vi "AerotechController.vi"() -> ()   [LabVIEW 2009]
uses:
  Controls/AerotechState.ctl
  Controls/AerotechCommand.ctl
  Controls/AerotechTarget.ctl
  Controls/AerotechScope.ctl
panel:
  out "Position error":dbl
  in  "Track threshold":dbl=5e-05
  in  "Gain [/s]":dbl=0.5
  out "Position":dbl
  out "State":T1
  in  "PROCESS":string="AEROTECH"
  in  "lpsParam":path=path "C:/OhanaOS/Instruments/Aerotech/Data/122764-A-1-1.prm"
  in  "lpsFirm":path=path "C:/u500/mmi/U500pci.jwp"
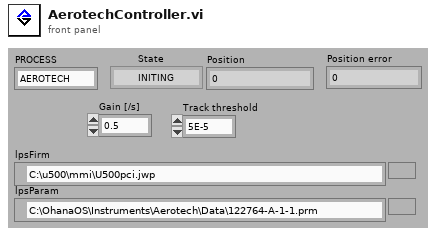
[diagram p1: front panel]
types:
  T1 = typedef "AerotechState.ctl" = enum16{"INITING", "IDLING", "SLEWING", "TRACKING", "MOVING", "HOMING", "STOPPING", "RECORDING"}
  T2 = typedef "AerotechCommand.ctl" = enum16{"TRACK", "POSITION", "STOP", "HOME", "QUIT", "RECORD"}
  T3 = typedef "AerotechSynchro.ctl" = cluster{"Command":refnum<queue>, "State":refnum<notifier>, "Target":refnum<notifier>, "Actual":refnum<notifier>, "Scope":refnum<notifier>}
  T4 = typedef "AerotechTarget.ctl" = cluster{"Time":timestamp, "Position":dbl, "Velocity":dbl}
  T5 = typedef "AerotechScope.ctl" = cluster{"First element":i32, "Buffer":i32[]}
  T6 = enum8{"Kill, clear memory", "Feedback Actual velocity data", "Feedback Command velocity data", "Feedback Auxiliary data", "Set time base (ms)", "Enable Tracking", "Stop Tracking, but keep data", "Set # of samples [1-2500]", "Set auxiliary sample type", "Feedback Auto tune Velocity", "Feedback Auto tune Torque"}
  T7 = cluster{"Position error":bool, "RMS current error":bool, "Integral error":bool, "Hardware limit +":bool, "Hardware limit -":bool, "Software limit +":bool, "Software limit -":bool, "Driver fault":bool, "Feedback device error":bool, "Global abort active":bool, "Velocity error":bool, "Feedrate > max setting error":bool, "Emergency stop":bool, "Driver interlock open":bool}
  T8 = cluster{"Axis 1 active":bool, "Axis 2 active":bool, "Axis 3 active":bool, "Axis 4 active":bool, "Axis 1 not in position":bool, "Axis 2 not in position":bool, "Axis 3 not in position":bool, "Axis 4 not in position":bool, "Plane 1 comm. busy":bool, "Plane 2 comm. busy":bool, "Plane 4 comm. busy":bool, "Plane 3 comm. busy":bool, "Queue 1 buffer not empty":bool, "Queue 2 buffer not empty":bool, "Queue 3 buffer not empty":bool, "Queue 4 buffer not empty":bool, "Plane 1 halted":bool, "Plane 2 halted":bool, "Plane 3 halted":bool, "Plane 4 halted":bool, "Global abort active":bool, "Feedhold active":bool, "PC Bus Interrupt high":bool, "Not ready for next command":bool}
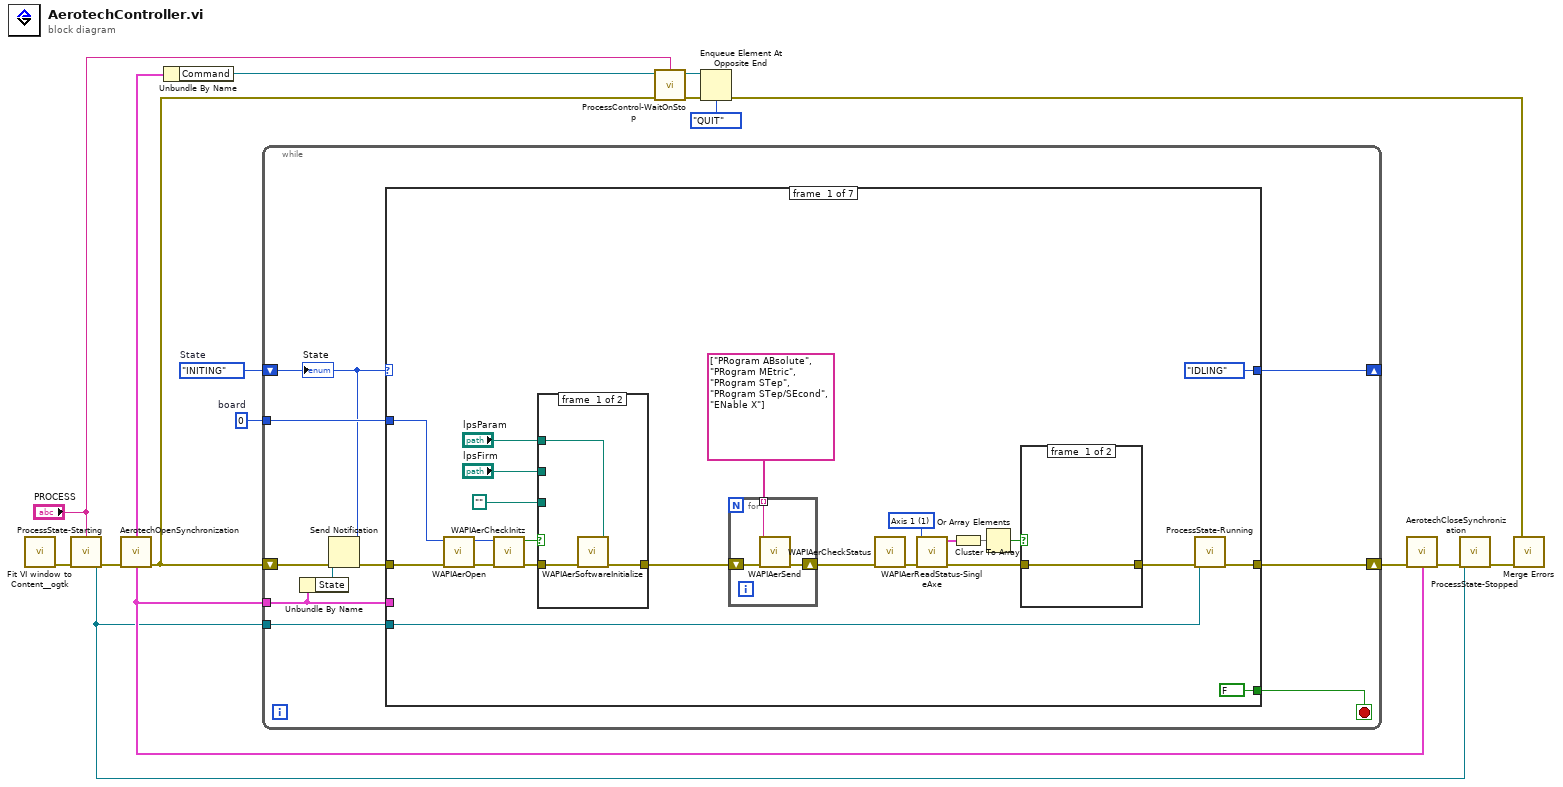
[diagram p0: block diagram]
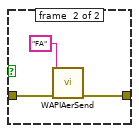
[diagram p2: hidden frame]
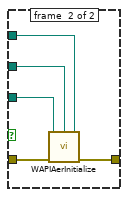
[diagram p3: hidden frame]
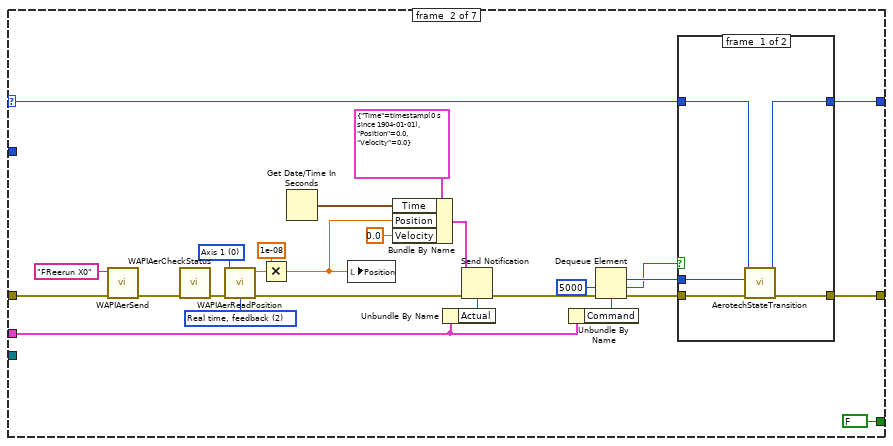
[diagram p4: hidden frame]
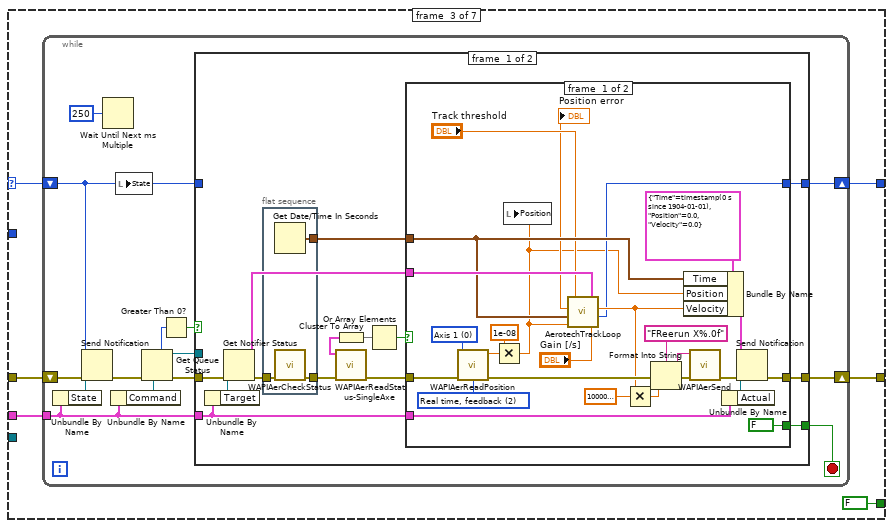
[diagram p6: hidden frame]
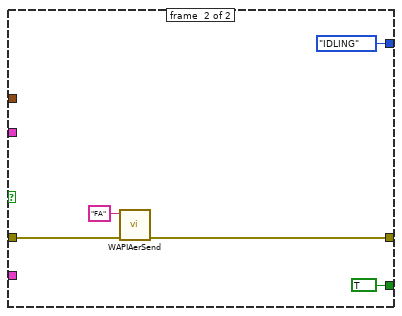
[diagram p7: hidden frame]
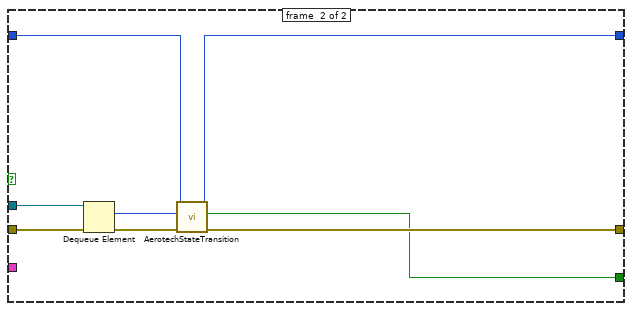
[diagram p8: hidden frame]
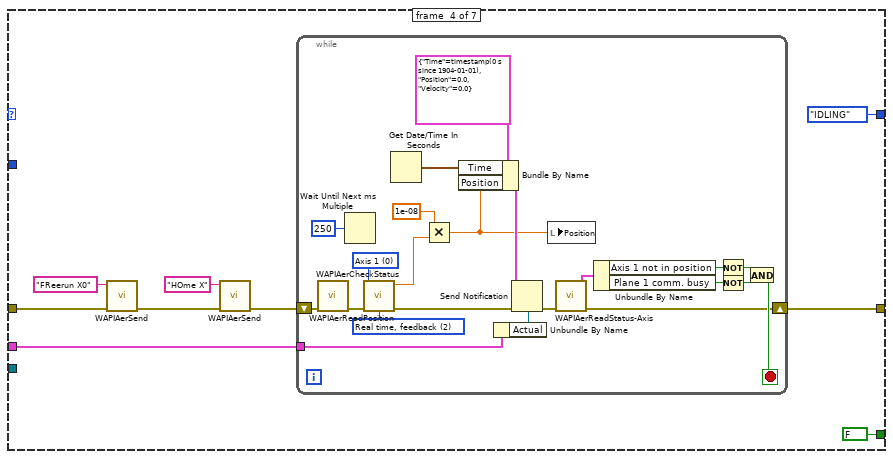
[diagram p9: hidden frame]
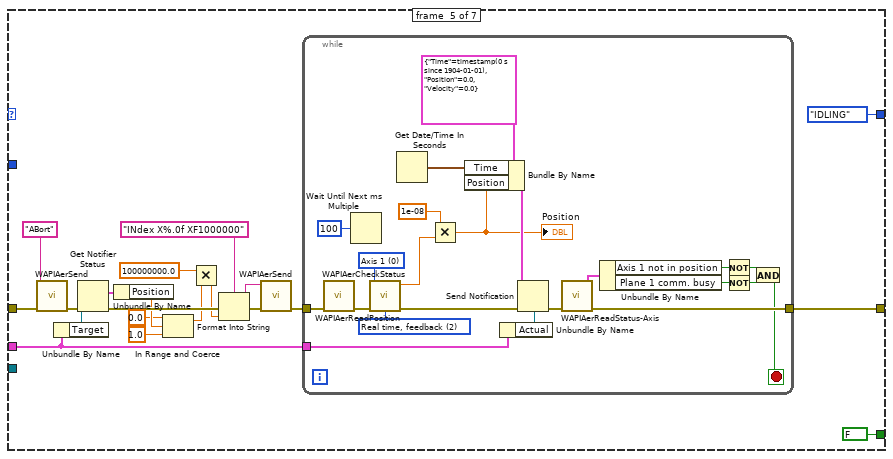
[diagram p10: hidden frame]
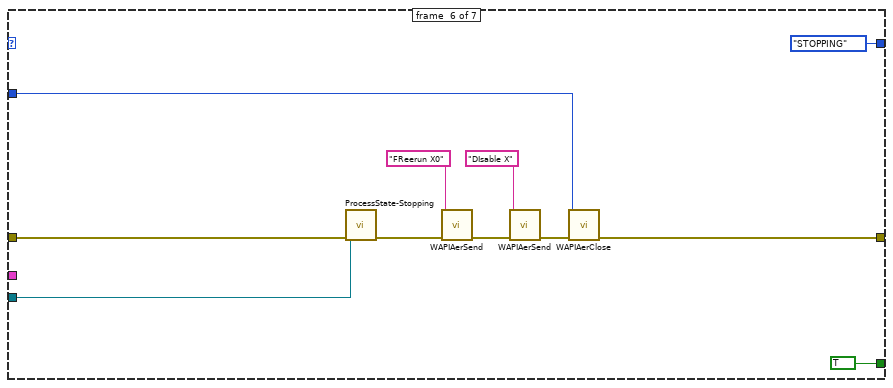
[diagram p11: hidden frame]
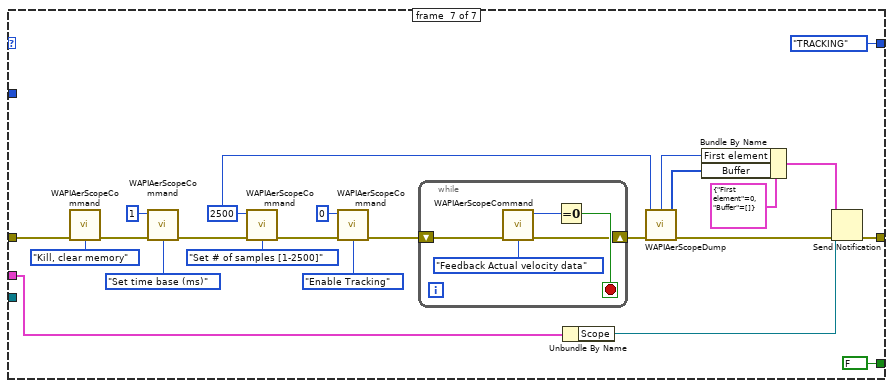
[diagram p12: hidden frame]
diagram:
  w13 = i16 0  # board
  w15 = AerotechState."INITING"  # State
  n1 = call <userlib>:"Fit VI window to Content__ogtk.vi"() -> ("error out"=w14:errorcluster)  [unwired: 6 in, 1 out]
  n2 = call "ProcessState-Starting.vi"("PROCESS"="PROCESS", "error in (no error)"=w14) -> ("ProcessStateNotifier"=w1:refnum<notifier>, "error in (no error)"=w12:errorcluster)  [unwired: 6 in]
  n3 = call "AerotechOpenSynchronization.vi"("error in (no error)"=w12) -> ("Synchro"=w2:T3, "error out"=w11:errorcluster)  [unwired: 7 in]
  n4 = Unbundle By Name(w2) -> ("Command"=w5:refnum<queue>)
  n5 = while {
    shift-right: [w23] -> _
    shift-left: w15 -> [w18]
    shift-right: [w25] -> w4
    shift-left: w11 -> [w20]
    tunnel: w13 -> [w21]
    tunnel: w2 -> [w16]
    tunnel: w1 -> [w24]
    stop <- w22 stop-if-true
    n6 = Unbundle By Name(w16) -> ("State"=w17:refnum<notifier>)
    n7 = Send Notification(notification=w18, notifier=w17, error in (no error)=w20) -> (error out=w19:errorcluster)  [unwired: 1 out]
    n8 = case shown="\"RECORDING\"" w18 {
      selector: w18 -> [_ w84 w98 _ _ _ _]
      tunnel: [w42 w86 w96 w173 w222 w251 w262] -> w25
      tunnel: w19 -> [w43 w82 w101 w176 w210 w254 w266]
      tunnel: w24 -> [w41 _ _ _ _ w253 _]
      tunnel: [AerotechState."IDLING" ("State") w83 w97 AerotechState."IDLING" ("State") AerotechState."IDLING" ("State") AerotechState."STOPPING" ("State") AerotechState."TRACKING" ("State")] -> w23
      tunnel: [FALSE FALSE FALSE FALSE FALSE TRUE FALSE] -> w22
      tunnel: w21 -> [w39 _ _ _ _ w252 _]
      tunnel: w16 -> [_ w79 w99 w172 w207 _ w259]
      frame #0 {
        w31 = i16 1 items=["Axis 1"=1, "Axis 2"=2, "Axis 3"=3, "Axis 4"=4] ("nAxis")
        n9 = call "WAPIAerOpen.vi"("error in (no error)"=w43, "board"=w39) -> ("error out"=w47:errorcluster)  [unwired: 9 in]
        n10 = call "WAPIAerCheckInitz.vi"("board"=w39, "error in (no error)"=w47) -> ("result"=w34:bool, "error out"=w46:errorcluster)  [unwired: 6 in]
        n11 = case shown="True" w34 {
          tunnel: w46 -> [w57 w62]
          tunnel: "lpsParam" -> [w55 w61]
          tunnel: "lpsFirm" -> [_ w60]
          tunnel: path "" -> [_ w59]
          tunnel: [w56 w58] -> w36
          frame #0 {
            n12 = call "WAPIAerSoftwareInitialize.vi"("lpsParam"=w55, "error in (no error)"=w57) -> ("error out"=w56:errorcluster)  [unwired: 7 in]
          }
          frame #1 {
            n13 = call "WAPIAerInitialize.vi"("lpsParam"=w61, "lpsFirm"=w60, "lpsConfig"=w59, "error in (no error)"=w62) -> ("error out"=w58:errorcluster)  [unwired: 5 in]
          }
        }
        n14 = for {
          shift-right: [w53] -> w33
          shift-left: w36 -> [w54]
          tunnel: string[] ["PRogram ABsolute", "PRogram MEtric", "PRogram STep", "PRogram STep/SEcond", "ENable X"] -> [w52] mode=indexing
          n15 = call "WAPIAerSend.vi"("error in (no error)"=w54, "lpsCmd"=w52) -> ("error out"=w53:errorcluster)  [unwired: 9 in]
        }
        n16 = call "WAPIAerCheckStatus.vi"("error in (no error)"=w33) -> ("error out"=w32:errorcluster)  [unwired: 8 in]
        n17 = call "WAPIAerReadStatus-SingleAxe.vi"("nAxis"=w31, "error in (no error)"=w32) -> ("Axis status"=w30:T7, "error out"=w27:errorcluster)  [unwired: 6 in]
        n18 = Cluster To Array(cluster=w30) -> (array=w28:bool[])
        n19 = Or Array Elements(Boolean array=w28) -> (logical OR=w29:bool)
        n20 = case shown="False" w29 {
          tunnel: w27 -> [w48 w51]
          tunnel: [w48 w49] -> w26
          frame #0 {
          }
          frame #1 {
            n21 = call "WAPIAerSend.vi"("error in (no error)"=w51, "lpsCmd"="FA") -> ("error out"=w49:errorcluster)  [unwired: 9 in]
          }
        }
        n22 = call "ProcessState-Running.vi"("ProcessStateNotifier in"=w41, "error in (no error)"=w26) -> ("error out"=w42:errorcluster)  [unwired: 6 in, 1 out]
      }
      frame #1 {
        w72 = i16 2 items=["Relative, commanded, not real time", "Absolute, commanded, not real time", "Real time, feedback", "Real time, commanded"] ("nType")
        w70 = i16 0 items=["Axis 1", "Axis 2", "Axis 3", "Axis 4"] ("nAxis")
        n23 = call "WAPIAerSend.vi"("error in (no error)"=w82, "lpsCmd"="FReerun X0") -> ("error out"=w69:errorcluster)  [unwired: 9 in]
        n24 = call "WAPIAerCheckStatus.vi"("error in (no error)"=w69) -> ("error out"=w73:errorcluster)  [unwired: 8 in]
        n25 = call "WAPIAerReadPosition.vi"("nAxis"=w70, "nType"=w72, "error in (no error)"=w73) -> ("Position"=w71:dbl, "error out"=w68:errorcluster)  [unwired: 5 in]
        n26 = Multiply(x=1e-08 ("y"), y=w71) -> (x*y=w63:dbl)
        n27 = Get Date/Time In Seconds() -> (seconds since 1Jan1904=w74:timestamp)
        n28 = local write "Position"(w63) -> ()
        n29 = Bundle By Name(cluster=T4 {"Time"=timestamp(0 s since 1904-01-01), "Position"=0.0, "Velocity"=0.0} ("notification"), "Time"=w74, "Position"=w63, "Velocity"=0.0) -> (w77:T4)
        n30 = Unbundle By Name(w79) -> ("Actual"=w76:refnum<notifier>)
        n31 = Send Notification(notification=w77, notifier=w76, error in (no error)=w68) -> (error out=w80:errorcluster)  [unwired: 1 out]
        n32 = Unbundle By Name(w79) -> ("Command"=w75:refnum<queue>)
        n33 = Dequeue Element(queue=w75, timeout in ms (-1)=5000, error in (no error)=w80) -> (element=w85:T2, timed out?=w64:bool, error out=w87:errorcluster)  [unwired: 1 out]
        n34 = case shown="True" w64 {
          tunnel: w87 -> [w93 w94]
          tunnel: [w92 w94] -> w86
          tunnel: w85 -> [w91 _]
          tunnel: w84 -> [w90 w95]
          tunnel: [w89 w95] -> w83
          frame #0 {
            n35 = call "AerotechStateTransition.vi"("error in (no error)"=w93, "Command"=w91, "State In"=w90) -> ("error out"=w92:errorcluster, "State Out"=w89:T1)  [unwired: 5 in, 1 out]
          }
          frame #1 {
          }
        }
      }
      frame #2 {
        n36 = while {
          tunnel: w99 -> [w106]
          shift-right: [w110] -> w97
          shift-left: w98 -> [w103]
          shift-right: [w109] -> w96
          shift-left: w101 -> [w105]
          stop <- w102 stop-if-true
          n37 = Unbundle By Name(w106) -> ("State"=w107:refnum<notifier>)
          n38 = Send Notification(notification=w103, notifier=w107, error in (no error)=w105) -> (error out=w104:errorcluster)  [unwired: 1 out]
          n39 = Wait Until Next ms Multiple(millisecond multiple=u32 250) -> ()  [unwired: 1 out]
          n40 = Unbundle By Name(w106) -> ("Command"=w115:refnum<queue>)
          n41 = local write "State"(w103) -> ()
          n42 = Get Queue Status(queue=w115, error in (no error)=w104) -> (queue out=w111:refnum<queue>, error out=w112:errorcluster, # elements in queue=w114:i32)  [unwired: 1 in, 5 out]
          n43 = Greater Than 0?(x=w114) -> (x > 0?=w113:bool)
          n44 = case shown="True" w113 {
            tunnel: w112 -> [w129 w171]
            tunnel: w111 -> [_ w170]
            tunnel: w103 -> [_ w167]
            tunnel: [w122 w166] -> w110
            tunnel: [w124 w165] -> w109
            tunnel: w106 -> [w125 _]
            tunnel: [w116 w164] -> w102
            frame #0 {
              n45 = Unbundle By Name(w125) -> ("Target"=w128:refnum<notifier>)
              n46 = Get Notifier Status(notifier=w128, error in (no error)=w129) -> (current notification=w126:T4, error out=w127:errorcluster)  [unwired: 3 out]
              n47 = flat-sequence {
                tunnel: w127 -> [w163]
                tunnel: [w162] -> w123
                tunnel: [w161] -> w119
                frame #0 {
                  n48 = Get Date/Time In Seconds() -> (seconds since 1Jan1904=w162:timestamp)
                  n49 = call "WAPIAerCheckStatus.vi"("error in (no error)"=w163) -> ("error out"=w161:errorcluster)  [unwired: 8 in]
                }
              }
              n50 = call "WAPIAerReadStatus-SingleAxe.vi"("error in (no error)"=w119) -> ("Axis status"=w120:T7, "error out"=w118:errorcluster)  [unwired: 7 in]
              n51 = Cluster To Array(cluster=w120) -> (array=w121:bool[])
              n52 = Or Array Elements(Boolean array=w121) -> (logical OR=w117:bool)
              n53 = case shown="False" w117 {
                tunnel: w126 -> [w152 _]
                tunnel: w125 -> [w146 _]
                tunnel: [w144 w158] -> w124
                tunnel: w123 -> [w140 _]
                tunnel: [w134 AerotechState."IDLING" ("State")] -> w122
                tunnel: w118 -> [w131 w159]
                tunnel: [FALSE ("Transition?") TRUE ("Transition?")] -> w116
                frame #0 {
                  w155 = i16 2 items=["Relative, commanded, not real time", "Absolute, commanded, not real time", "Real time, feedback", "Real time, commanded"] ("nType")
                  w136 = i16 0 items=["Axis 1", "Axis 2", "Axis 3", "Axis 4"] ("nAxis")
                  n54 = call "WAPIAerReadPosition.vi"("nAxis"=w136, "nType"=w155, "error in (no error)"=w131) -> ("Position"=w154:dbl, "error out"=w150:errorcluster)  [unwired: 5 in]
                  n55 = Multiply(x=1e-08 ("y"), y=w154) -> (x*y=w132:dbl)
                  n56 = local write "Position"(w132) -> ()
                  n57 = call "AerotechTrackLoop.vi"("Gain [/s]"="Gain [/s]", "AEROTECH.TARGET"=w152, "Aerotech Position"=w132, "Aerotech Time"=w140, "Track threshold"="Track threshold") -> ("State"=w134:T1, "Aerotech Velocity"=w137:dbl, "Position error"=→"Position error":dbl)
                  n58 = Multiply(x=w137, y=100000000.0) -> (x*y=w139:dbl)
                  n59 = Format Into String(format string="FReerun X%.0f" ("lpsCmd"), error in=w150, w139) -> (resulting string=w148:string, error out=w149:errorcluster)  [unwired: 1 in]
                  n60 = Bundle By Name(cluster=T4 {"Time"=timestamp(0 s since 1904-01-01), "Position"=0.0, "Velocity"=0.0} ("notification"), "Time"=w140, "Position"=w132, "Velocity"=w137) -> (w141:T4)
                  n61 = call "WAPIAerSend.vi"("error in (no error)"=w149, "lpsCmd"=w148) -> ("error out"=w145:errorcluster)  [unwired: 9 in]
                  n62 = Unbundle By Name(w146) -> ("Actual"=w143:refnum<notifier>)
                  n63 = Send Notification(notification=w141, notifier=w143, error in (no error)=w145) -> (error out=w144:errorcluster)  [unwired: 1 out]
                }
                frame #1 {
                  n64 = call "WAPIAerSend.vi"("error in (no error)"=w159, "lpsCmd"="FA") -> ("error out"=w158:errorcluster)  [unwired: 9 in]
                }
              }
            }
            frame #1 {
              n65 = Dequeue Element(queue=w170, error in (no error)=w171) -> (element=w168:T2, error out=w169:errorcluster)  [unwired: 1 in, 2 out]
              n66 = call "AerotechStateTransition.vi"("error in (no error)"=w169, "Command"=w168, "State In"=w167) -> ("error out"=w165:errorcluster, "Transition?"=w164:bool, "State Out"=w166:T1)  [unwired: 5 in]
            }
          }
        }
      }
      frame #3 {
        n67 = call "WAPIAerSend.vi"("error in (no error)"=w176, "lpsCmd"="FReerun X0") -> ("error out"=w175:errorcluster)  [unwired: 9 in]
        n68 = call "WAPIAerSend.vi"("error in (no error)"=w175, "lpsCmd"="HOme X") -> ("error out"=w174:errorcluster)  [unwired: 9 in]
        n69 = while {
          tunnel: w172 -> [w189]
          shift-right: [w182] -> w173
          shift-left: w174 -> [w197]
          stop <- w190 stop-if-true
          w194 = i16 2 items=["Relative, commanded, not real time", "Absolute, commanded, not real time", "Real time, feedback", "Real time, commanded"] ("nType")
          w193 = i16 0 items=["Axis 1", "Axis 2", "Axis 3", "Axis 4"] ("nAxis")
          n70 = call "WAPIAerCheckStatus.vi"("error in (no error)"=w197) -> ("error out"=w196:errorcluster)  [unwired: 8 in]
          n71 = Wait Until Next ms Multiple(millisecond multiple=u32 250) -> ()  [unwired: 1 out]
          n72 = call "WAPIAerReadPosition.vi"("nAxis"=w193, "nType"=w194, "error in (no error)"=w196) -> ("Position"=w192:dbl, "error out"=w188:errorcluster)  [unwired: 5 in]
          n73 = Get Date/Time In Seconds() -> (seconds since 1Jan1904=w183:timestamp)
          n74 = Multiply(x=1e-08, y=w192) -> (x*y=w181:dbl)
          n75 = Bundle By Name(cluster=T4 {"Time"=timestamp(0 s since 1904-01-01), "Position"=0.0, "Velocity"=0.0} ("notification"), "Time"=w183, "Position"=w181) -> (w184:T4)
          n76 = Unbundle By Name(w189) -> ("Actual"=w186:refnum<notifier>)
          n77 = Send Notification(notification=w184, notifier=w186, error in (no error)=w188) -> (error out=w187:errorcluster)  [unwired: 1 out]
          n78 = local write "Position"(w181) -> ()
          n79 = call "WAPIAerReadStatus-Axis.vi"("error in (no error)"=w187) -> ("Axis/Plane/Queue status"=w202:T8, "error out"=w182:errorcluster)  [unwired: 7 in]
          n80 = Unbundle By Name(w202) -> ("Axis 1 not in position"=w201:bool, "Plane 1 comm. busy"=w200:bool)
          n81 = Not(x=w201) -> (.not. x?=w199:bool)
          n82 = Not(x=w200) -> (.not. x?=w198:bool)
          n83 = And(x=w199, y=w198) -> (x .and. y?=w190:bool)
        }
      }
      frame #4 {
        n84 = call "WAPIAerSend.vi"("error in (no error)"=w210, "lpsCmd"="ABort") -> ("error out"=w209:errorcluster)  [unwired: 9 in]
        n85 = Unbundle By Name(w207) -> ("Target"=w219:refnum<notifier>)
        n86 = Get Notifier Status(notifier=w219, error in (no error)=w209) -> (current notification=w218:T4, error out=w216:errorcluster)  [unwired: 3 out]
        n87 = Unbundle By Name(w218) -> ("Position"=w206:dbl)
        n88 = In Range and Coerce(upper limit=0.0, x=w206, lower limit=1.0) -> (coerced(x)=w205:dbl)  [unwired: 1 out]
        n89 = Multiply(x=100000000.0, y=w205) -> (x*y=w213:dbl)
        n90 = Format Into String(format string="INdex X%.0f XF1000000" ("lpsCmd"), error in=w216, w213) -> (resulting string=w212:string, error out=w215:errorcluster)  [unwired: 1 in]
        n91 = call "WAPIAerSend.vi"("error in (no error)"=w215, "lpsCmd"=w212) -> ("error out"=w211:errorcluster)  [unwired: 9 in]
        n92 = while {
          tunnel: w211 -> [w239]
          tunnel: [w237] -> w222
          tunnel: w207 -> [w230]
          stop <- w231 stop-if-true
          w235 = i16 2 items=["Relative, commanded, not real time", "Absolute, commanded, not real time", "Real time, feedback", "Real time, commanded"] ("nType")
          w234 = i16 0 items=["Axis 1", "Axis 2", "Axis 3", "Axis 4"] ("nAxis")
          n93 = call "WAPIAerCheckStatus.vi"("error in (no error)"=w239) -> ("error out"=w238:errorcluster)  [unwired: 8 in]
          n94 = Wait Until Next ms Multiple(millisecond multiple=u32 100) -> ()  [unwired: 1 out]
          n95 = call "WAPIAerReadPosition.vi"("nAxis"=w234, "nType"=w235, "error in (no error)"=w238) -> ("Position"=w233:dbl, "error out"=w229:errorcluster)  [unwired: 5 in]
          n96 = Get Date/Time In Seconds() -> (seconds since 1Jan1904=w224:timestamp)
          n97 = Multiply(x=1e-08, y=w233) -> (x*y=w223:dbl)
          "Position" <- w223
          n98 = Bundle By Name(cluster=T4 {"Time"=timestamp(0 s since 1904-01-01), "Position"=0.0, "Velocity"=0.0} ("notification"), "Time"=w224, "Position"=w223) -> (w225:T4)
          n99 = Unbundle By Name(w230) -> ("Actual"=w227:refnum<notifier>)
          n100 = Send Notification(notification=w225, notifier=w227, error in (no error)=w229) -> (error out=w228:errorcluster)  [unwired: 1 out]
          n101 = call "WAPIAerReadStatus-Axis.vi"("error in (no error)"=w228) -> ("Axis/Plane/Queue status"=w244:T8, "error out"=w237:errorcluster)  [unwired: 7 in]
          n102 = Unbundle By Name(w244) -> ("Axis 1 not in position"=w243:bool, "Plane 1 comm. busy"=w242:bool)
          n103 = Not(x=w243) -> (.not. x?=w241:bool)
          n104 = Not(x=w242) -> (.not. x?=w240:bool)
          n105 = And(x=w241, y=w240) -> (x .and. y?=w231:bool)
        }
      }
      frame #5 {
        n106 = call "ProcessState-Stopping.vi"("ProcessStateNotifier in"=w253, "error in (no error)"=w254) -> ("error out"=w248:errorcluster)  [unwired: 6 in, 1 out]
        n107 = call "WAPIAerSend.vi"("error in (no error)"=w248, "lpsCmd"="FReerun X0") -> ("error out"=w246:errorcluster)  [unwired: 9 in]
        n108 = call "WAPIAerSend.vi"("error in (no error)"=w246, "lpsCmd"="DIsable X") -> ("error out"=w245:errorcluster)  [unwired: 9 in]
        n109 = call "WAPIAerClose.vi"("error in (no error)"=w245, "board"=w252) -> ("error out"=w251:errorcluster)  [unwired: 9 in]
      }
      frame #6 {
        w272 = u16 2500 ("data")
        n110 = call "WAPIAerScopeCommand.vi"("cmd"=T6."Kill, clear memory", "error in (no error)"=w266) -> ("error out"=w273:errorcluster)  [unwired: 6 in, 1 out]
        n111 = call "WAPIAerScopeCommand.vi"("data"=u16 1, "cmd"=T6."Set time base (ms)", "error in (no error)"=w273) -> ("error out"=w268:errorcluster)  [unwired: 5 in, 1 out]
        n112 = call "WAPIAerScopeCommand.vi"("data"=w272, "cmd"=T6."Set # of samples [1-2500]", "error in (no error)"=w268) -> ("error out"=w270:errorcluster)  [unwired: 5 in, 1 out]
        n113 = call "WAPIAerScopeCommand.vi"("data"=u16 0, "cmd"=T6."Enable Tracking", "error in (no error)"=w270) -> ("error out"=w274:errorcluster)  [unwired: 5 in, 1 out]
        n114 = while {
          shift-right: [w280] -> w271
          shift-left: w274 -> [w283]
          stop <- w281 stop-if-true
          n115 = call "WAPIAerScopeCommand.vi"("cmd"=T6."Feedback Actual velocity data", "error in (no error)"=w283) -> ("count"=w282:i32, "error out"=w280:errorcluster)  [unwired: 6 in]
          n116 = Equal To 0?(x=w282) -> (x = 0?=w281:bool)
        }
        n117 = Unbundle By Name(w259) -> ("Scope"=w261:refnum<notifier>)
        n118 = call "WAPIAerScopeDump.vi"("count"=w272, "error in (no error)"=w271) -> ("scopebuf"=w258:i32[], "firstdata"=w257:i32, "error out"=w263:errorcluster)  [unwired: 5 in]
        n119 = Bundle By Name(cluster=T5 {"First element"=0, "Buffer"=[]} ("notification"), "First element"=w257, "Buffer"=w258) -> (w256:T5)
        n120 = Send Notification(notification=w256, notifier=w261, error in (no error)=w263) -> (error out=w262:errorcluster)  [unwired: 1 out]
      }
    }
    "State" <- w18
  }
  n121 = call "ProcessControl-WaitOnStop.vi"("PROCESS"="PROCESS", "error out"=w11) -> ("error in"=w10:errorcluster)  [unwired: 7 in]
  n122 = Enqueue Element At Opposite End(queue=w5, element=AerotechCommand."QUIT", error in (no error)=w10) -> (error out=w6:errorcluster)  [unwired: 1 in, 2 out]
  n123 = call "AerotechCloseSynchronization.vi"("Synchro"=w2, "error in (no error)"=w4) -> ("error out"=w3:errorcluster)  [unwired: 7 in]
  n124 = call "ProcessState-Stopped.vi"("ProcessStateNotifier in"=w1, "error in (no error)"=w3) -> ("error out"=w7:errorcluster)  [unwired: 7 in]
  n125 = call <vilib>:"Merge Errors.vi"("error in 3 (no error)"=w7, "error in 1 (no error)"=w6) -> ()  [unwired: 5 in, 1 out]
